vi "Run.vi"(8 "error in (no error)":errorcluster, 11 "Channel Pub in":refnum<class "Channel Pub.lvclass">) -> (0 "error out":errorcluster, 3 "Channel Pub out":refnum<class "Channel Pub.lvclass">)   [LabVIEW 2018, in "Channel Pub.lvclass"]
uses:
  Channel Pub.lvclass
  Communication Channel/Communication Channel.lvclass
  State Machine/State Machine.lvclass
  Socket/Socket.lvclass
  RxTx/RxTx.lvclass
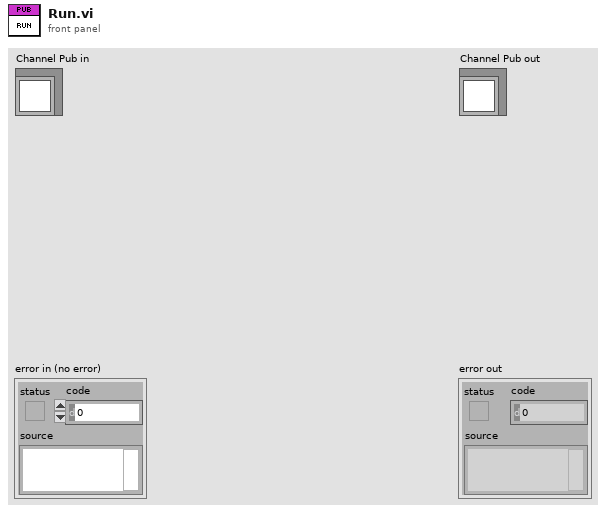
[diagram p1: front panel]
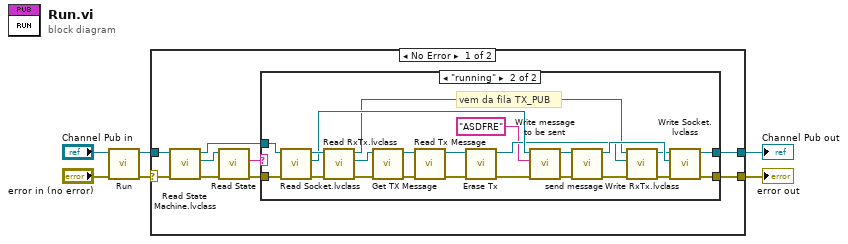
[diagram p0: block diagram]
diagram:
  n1 = call-parent "Run.vi"("error in (no error)"="error in (no error)", "Communication Channel in"="Channel Pub in") -> ("error out"=w4:errorcluster, "Communication Channel out"=w3:refnum<class "Channel Pub.lvclass">)  [unwired: 8 in]
  n2 = case shown="No Error" w4 {
    selector: w4 -> [w14 w41]
    tunnel: w3 -> [w15 w42]
    tunnel: [w8 w42] -> w2
    tunnel: [w9 w41] -> w1
    frame No Error {
      n3 = call-dynamic "Read State Machine.lvclass.vi"("error in (no error)"=w14, "Communication Channel in"=w15) -> ("error out"=w13:errorcluster, "State Machine.lvclass"=w10:refnum<class "State Machine.lvclass">, "Communication Channel out"=w11:refnum<class "Channel Pub.lvclass">)  [unwired: 7 in]
      n4 = call-dynamic "Read State.vi"("error in (no error)"=w13, "State Machine in"=w10) -> ("error out"=w7:errorcluster, "State"=w12:string)  [unwired: 7 in, 1 out]
      n5 = case shown="\"running\"" w12 {
        tunnel: w11 -> [w17 w34]
        tunnel: [w17 w27] -> w8
        tunnel: [w16 w24] -> w9
        tunnel: w7 -> [w16 w23]
        frame Default {
        }
        frame "running" {
          # "vem da fila TX_PUB"
          n6 = call-dynamic "Read Socket.lvclass.vi"("error in (no error)"=w23, "Communication Channel in"=w34) -> ("error out"=w30:errorcluster, "Socket.lvclass"=w32:refnum<class "Socket.lvclass">, "Communication Channel out"=w33:refnum<class "Channel Pub.lvclass">)  [unwired: 7 in]
          n7 = call-dynamic "Read RxTx.lvclass.vi"("error in (no error)"=w30, "Communication Channel in"=w33) -> ("error out"=w35:errorcluster, "RxTx.lvclass"=w36:refnum<class "RxTx.lvclass">, "Communication Channel out"=w29:refnum<class "Channel Pub.lvclass">)  [unwired: 7 in]
          n8 = call "Get TX Message.vi"("error in (no error)"=w35, "RxTx in"=w36) -> ("error out"=w39:errorcluster, "RxTx out"=w40:refnum<class "RxTx.lvclass">)  [unwired: 7 in, 1 out]
          n9 = call "Read Tx Message.vi"("error in (no error)"=w39, "RxTx in"=w40) -> ("error out"=w22:errorcluster, "RxTx out"=w19:refnum<class "RxTx.lvclass">)  [unwired: 7 in, 1 out]
          n10 = call "Erase Tx.vi"("error in (no error)"=w22, "RxTx in"=w19) -> ("error out"=w21:errorcluster, "RxTx out"=w20:refnum<class "RxTx.lvclass">)  [unwired: 8 in]
          n11 = call-dynamic "Write message to be sent.vi"("error in (no error)"=w21, "message to be sent"="ASDFRE", "Socket in"=w32) -> ("error out"=w38:errorcluster, "Socket out"=w37:refnum<class "Socket.lvclass">)  [unwired: 7 in]
          n12 = call "send message.vi"("error in (no error)"=w38, "Socket in"=w37) -> ("error out"=w26:errorcluster, "Socket out"=w31:refnum<class "Socket.lvclass">)  [unwired: 8 in]
          n13 = call-dynamic "Write RxTx.lvclass.vi"("error in (no error)"=w26, "RxTx.lvclass"=w20, "Communication Channel in"=w29) -> ("error out"=w25:errorcluster, "Communication Channel out"=w28:refnum<class "Channel Pub.lvclass">)  [unwired: 7 in]
          n14 = call-dynamic "Write Socket.lvclass.vi"("error in (no error)"=w25, "Socket2.lvclass"=w31, "Communication Channel in"=w28) -> ("error out"=w24:errorcluster, "Communication Channel out"=w27:refnum<class "Channel Pub.lvclass">)  [unwired: 7 in]
        }
      }
    }
    frame Error {
    }
  }
  "Channel Pub out" <- w2
  "error out" <- w1
